vi "ESC_StdSci_Driver.vi"(10 "串口写数据包":T1={"包头"=170, "数据低8位"=0, "数据低高8位"=0, "数据类型"=0, "CRC余数"=0, "数据无效"=FALSE, "数据更新"=FALSE} {"包头" format="%02x"; "数据低8位" format="%02x"; "数据低高8位" format="%02x"; "数据类型" items=["VOID"]; "CRC余数" format="%02x"}, 11 "VISA资源名称":refnum<visa-resource-name>="COM1") -> (2 "串口读数据包":T1={"包头"=170, "数据低8位"=0, "数据低高8位"=0, "数据类型"=0, "CRC余数"=0, "数据无效"=FALSE, "数据更新"=FALSE} {"包头" format="%02x"; "数据低8位" format="%02x"; "数据低高8位" format="%02x"; "数据类型" items=["VOID"]; "CRC余数" format="%02x"}, 3 "串口读数据":i32[](array[numeric]) format="%04x", 4 "串口读缓存字符数":u32, 5 "串口缓存非空":bool, 7 "写数据更新":bool, 8 "串口写入数据包":T1={"包头"=170, "数据低8位"=0, "数据低高8位"=0, "数据类型"=0, "CRC余数"=0, "数据无效"=FALSE, "数据更新"=FALSE} {"包头" format="%02x"; "数据低8位" format="%02x"; "数据低高8位" format="%02x"; "数据类型" items=["VOID"]; "CRC余数" format="%02x"}, 9 "串口写入数据":string)   [LabVIEW 2015]
uses:
  SCI_DataPck.ctl
  SCI_DataType.ctl
  <vilib>/Instr/_visa.llb/VISA Configure Serial Port (Instr).vi
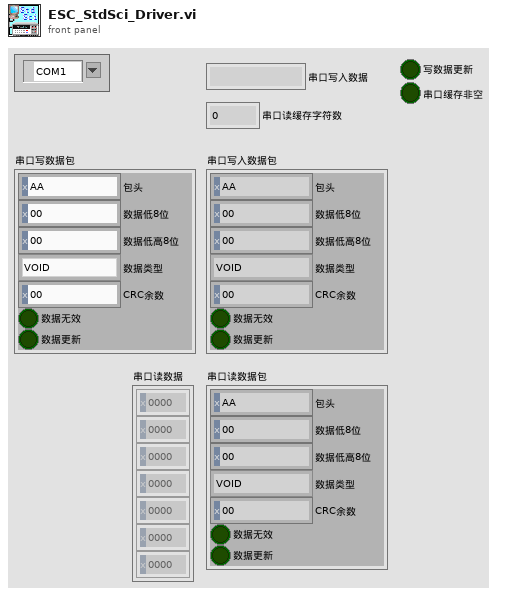
[diagram p1: front panel]
types:
  T1 = typedef "SCI_DataPck.ctl" = cluster{"包头":u16, "数据低8位":u16, "数据低高8位":u16, "数据类型":T2, "CRC余数":u16, "数据无效":bool, "数据更新":bool}
  T2 = typedef "SCI_DataType.ctl" = u16
  T3 = cluster{"波特率":u32, "数据比特":u16, "奇偶":enum16{"None", "Odd", "Even", "Mark", "Space"}, "停止位":u16, "流控制":u16}
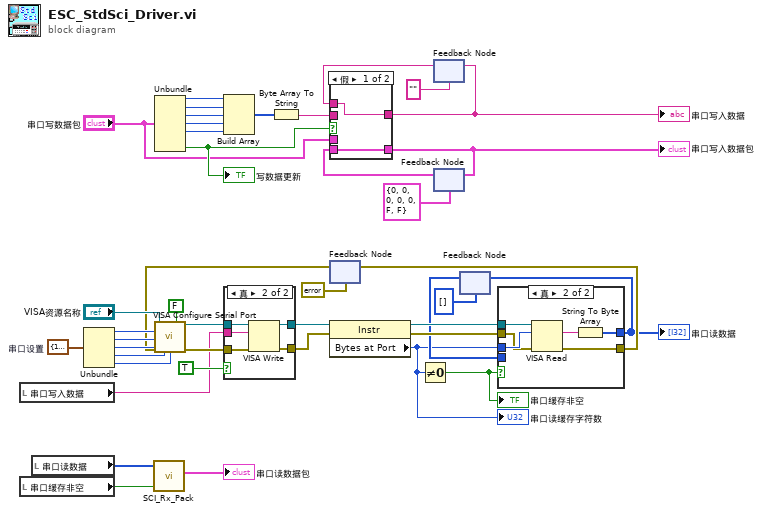
[diagram p0: block diagram]
diagram:
  w36 = T3 {"波特率"=115200, "数据比特"=8, "奇偶"=enum."None", "停止位"=10, "流控制"=0}  # 串口设置
  n1 = local read "串口写入数据"() -> (w1:string)
  n2 = local read "串口缓存非空"() -> (w26:bool)
  n3 = local read "串口读数据"() -> (w27:i32[])
  n4 = Unbundle(w36) -> ("波特率"=w41:u32, "数据比特"=w40:u16, "奇偶"=w39:enum16{"None", "Odd", "Even", "Mark", "Space"}, "停止位"=w38:u16, "流控制"=w37:u16)
  n5 = call "SCI_Rx_Pack.vi"("确认"=w26, "SCI RX数据块"=w27) -> ("SciPckOut"=→"串口读数据包":T1)  [unwired: 5 in, 1 out]
  n6 = Unbundle("串口写数据包") -> ("包头"=w23:u16, "数据低8位"=w22:u16, "数据低高8位"=w21:u16, "数据类型"=w20:T2, "CRC余数"=w19:u16, "数据更新"=w13:bool)  [unwired: 1 out]
  "写数据更新" <- w13
  n7 = Build Array(w23, w22, w21, w20, w19) -> (w18:T2[])
  n8 = Byte Array To String(unsigned byte array=w18) -> (string=w5:string)
  n9 = feedback #1(errorcluster {"status"=FALSE, "code"=0, "source"=""} ("error out")) -> (w14:errorcluster)
  n10 = call-poly "VISA Configure Serial Port"("VISA resource name"="VISA资源名称", "Enable Termination\nChar (T)"=FALSE, "baud rate (9600)"=w41, "data bits (8)"=w40, "parity (0:none)"=w39, "error in (no error)"=w14, "stop bits (10: 1 bit)"=w38, "flow control (0:none)"=w37) -> ("VISA resource name out"=w32:refnum<visa-resource-name>, "error out"=w35:errorcluster)  [unwired: 1 in, 5 out]
  n11 = case shown="真" TRUE {
    tunnel: w35 -> [w43 w49]
    tunnel: [w43 w48] -> w34
    tunnel: [w44 w47] -> w33
    tunnel: w32 -> [w44 w46]
    tunnel: w1 -> [_ w45]
    frame False {
    }
    frame True {
      n12 = VISA Write(VISA resource name=w46, write buffer=w45, error in (no error)=w49) -> (VISA resource name out=w47:refnum<visa-resource-name>, error out=w48:errorcluster)  [unwired: 1 out]
    }
  }
  n13 = property class="Instr"(reference=w33, error in=w34) -> (reference out=w31:refnum<visa-resource-name>, error out=w30:errorcluster, "Bytes at Port"=w9:u32)
  "串口读缓存字符数" <- w9
  n14 = Not Equal To 0?(x=w9) -> (x != 0?=w29:bool)
  "串口缓存非空" <- w29
  n15 = feedback #2("" ("string")) -> (w6:string)
  n16 = feedback #3(T1 {"包头"=0, "数据低8位"=0, "数据低高8位"=0, "数据类型"=0, "CRC余数"=0, "数据无效"=FALSE, "数据更新"=FALSE}) -> (w15:T1)
  n17 = case shown="假" w13 {
    tunnel: "串口写数据包" -> [_ w53]
    tunnel: [w51 w53] -> w16
    tunnel: w15 -> [w51 _]
    tunnel: w6 -> [w50 _]
    tunnel: [w50 w52] -> w2
    tunnel: w5 -> [_ w52]
    frame False {
    }
    frame True {
    }
  }
  "串口写入数据" <- w2
  "串口写入数据包" <- w16
  n18 = feedback-in #2(w2) -> ()
  n19 = feedback-in #3(w16) -> ()
  n20 = feedback #4(u8[] [] ("unsigned byte array")) -> (w10:u8[])
  n21 = case shown="真" w29 {
    tunnel: w10 -> [w55 _]
    tunnel: [w55 w58] -> w11
    tunnel: w31 -> [_ w60]
    tunnel: w9 -> [_ w59]
    tunnel: w30 -> [w54 w57]
    tunnel: [w54 w56] -> w25
    frame False {
    }
    frame True {
      n22 = VISA Read(VISA resource name=w60, byte count=w59, error in (no error)=w57) -> (read buffer=w61:string, error out=w56:errorcluster)  [unwired: 2 out]
      n23 = String To Byte Array(string=w61) -> (unsigned byte array=w58:u8[])
    }
  }
  "串口读数据" <- w11
  n24 = feedback-in #1(w25) -> ()
  n25 = feedback-in #4(w11) -> ()
